vi "SetControlsEnableDisableVisibleStates.vi"(8 "error in (no error)":errorcluster, 11 "Array":T1[](array[typedef])) -> (0 "error out":errorcluster)   [LabVIEW 2017]
doc: "This vi iterates through all controls registered in the given array and sets their enabled disables visible state to the stored values"
uses:
  Types/ControlAttributes.ctl
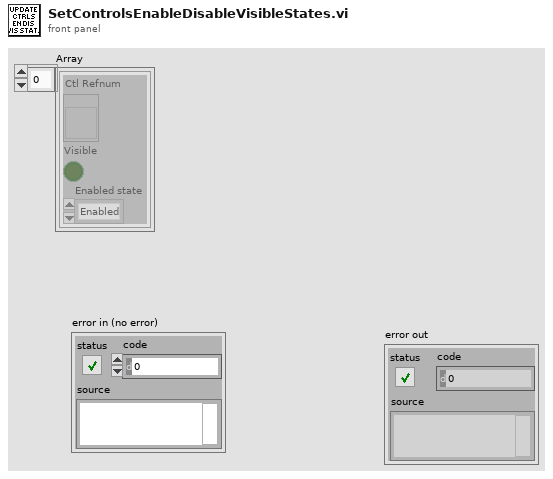
[diagram p1: front panel]
types:
  T1 = typedef "ControlAttributes.ctl" = cluster{"Ctl Refnum":refnum<vi>, "Visible":bool, "Enabled state":enum8{"Enabled", "Disabled", "Disabled and Grayed Out"}}
  T2 = enum8{"Enabled", "Disabled", "Disabled and Grayed Out"}
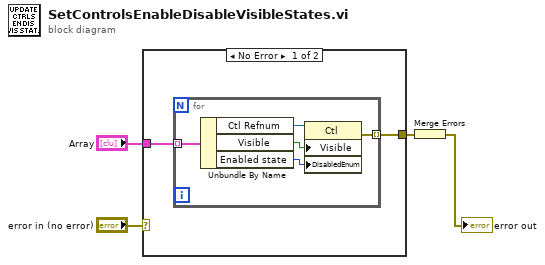
[diagram p0: block diagram]
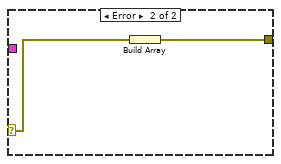
[diagram p2: hidden frame]
diagram:
  n1 = case shown="No Error" "error in (no error)" {
    selector: "error in (no error)" -> [_ w13]
    tunnel: [w6 w12] -> w4
    tunnel: "Array" -> [w5 _]
    frame No Error {
      n2 = for {
        tunnel: w5 -> [w11] mode=indexing
        tunnel: [w7] -> w6 mode=indexing
        n3 = Unbundle By Name(w11) -> ("Ctl Refnum"=w8:refnum<vi>, "Visible"=w10:bool, "Enabled state"=w9:T2)
        n4 = property class="Ctl"(reference=w8, "Visible"=w10, "DisabledEnum"=w9) -> (error out=w7:errorcluster)  [unwired: 1 in, 1 out]
      }
    }
    frame Error {
      n5 = Build Array(w13) -> (w12:errorcluster[])
    }
  }
  n6 = Merge Errors(w4) -> (→"error out":errorcluster)
